vi "Get Deploy Directories.vi"(7 "Subdirectory":string="Data Sharing Framework Core", 8 "error in (no error)":errorcluster, 11 "Target":T1) -> (0 "error out":errorcluster, 3 "Directories to Deploy To":path[](array[path]))   [LabVIEW 2017]
uses:
  Target Type.ctl
  Constants.vi
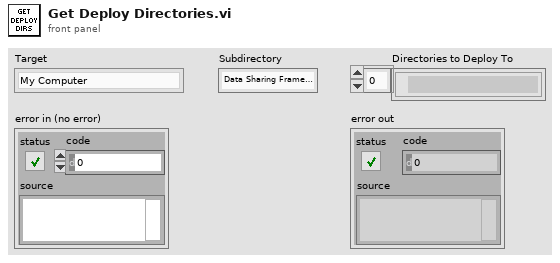
[diagram p1: front panel]
types:
  T1 = typedef "Target Type.ctl" = enum16{"My Computer", "Pharlap"}
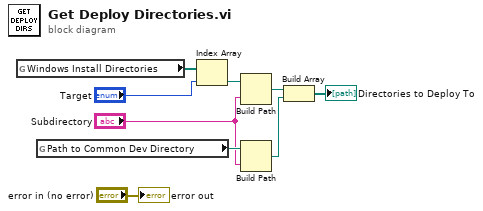
[diagram p0: block diagram]
diagram:
  n1 = global read "Constants.vi" "Windows Install Directories"() -> (w1:path[])
  n2 = global read "Constants.vi" "Path to Common Dev Directory"() -> (w7:path)
  n3 = Index Array(array=w1, index="Target") -> (element=w4:path)
  n4 = Build Path(base path=w4, name or relative path="Subdirectory") -> (appended path=w3:path)
  n5 = Build Path(base path=w7, name or relative path="Subdirectory") -> (appended path=w9:path)
  n6 = Build Array(w3, w9) -> (→"Directories to Deploy To":path[])
  "error out" <- "error in (no error)"
